vi "Get Device Model From Class Path.vi"(11 "MetaDataObj in":refnum<class "MetaDataObj.lvclass">) -> (1 "Dev Ethernet Port":string, 2 "Device Model Str":string, 3 "MetaDataObj Out":refnum<class "MetaDataObj.lvclass">)   [LabVIEW 2021, in "myRIOMetaDataObj.lvclass"]
uses:
  myRIOMetaDataObj.lvclass
  <resource>/dialog/NewProjectWizard/MetaDataObj/MetaDataObj.lvclass
  <resource>/dialog/NewProjectWizard/MetaDataObj/MetaDataObj.lvclass/MetaDataObj.ctl
  <resource>/dialog/NewProjectWizard/MetaDataObj/Accessors/Read Child Class Path.vi
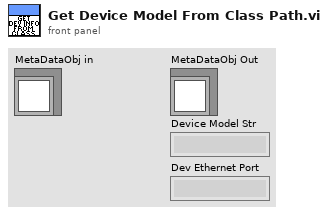
[diagram p1: front panel]
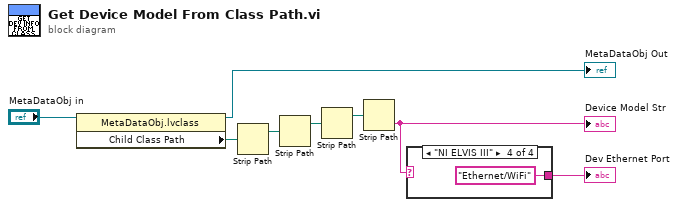
[diagram p0: block diagram]
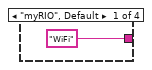
[diagram p2: hidden frame]
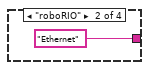
[diagram p3: hidden frame]
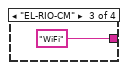
[diagram p4: hidden frame]
diagram:
  n1 = property class="MetaDataObj.lvclass"(reference="MetaDataObj in") -> (reference out=→"MetaDataObj Out":refnum<class "MetaDataObj.lvclass">, "Child Class Path"=w5:path)  [unwired: 1 in, 1 out]
  n2 = Strip Path(path=w5) -> (stripped path=w8:path)  [unwired: 1 out]
  n3 = Strip Path(path=w8) -> (stripped path=w7:path)  [unwired: 1 out]
  n4 = Strip Path(path=w7) -> (stripped path=w6:path)  [unwired: 1 out]
  n5 = Strip Path(path=w6) -> (name=w2:string)  [unwired: 1 out]
  "Device Model Str" <- w2
  n6 = case shown="\"NI ELVIS III\"" w2 {
    tunnel: ["WiFi" "Ethernet" "WiFi" "Ethernet/WiFi"] -> w1
    frame "myRIO", Default {
    }
    frame "roboRIO" {
    }
    frame "EL-RIO-CM" {
    }
    frame "NI ELVIS III" {
    }
  }
  "Dev Ethernet Port" <- w1
